vi "Text_without_format.vi"(1 "Input string":string) -> (0 "Output string":string)   [LabVIEW 2010]
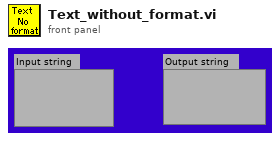
[diagram p1: front panel]
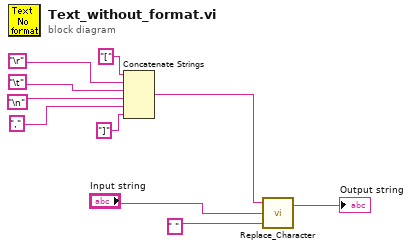
[diagram p0: block diagram]
diagram:
  n1 = Concatenate Strings("[" ("Substring"), "\r", "\t", "\n", ",", "]" ("Substring")) -> (w1:string)
  n2 = call "Replace_Character.vi"("Replace with"=" " ("After  Matched string"), "Input String"="Input string", "Search For"=w1) -> ("Output string"=→"Output string":string)  [unwired: 1 out]
